vi "setSlideState.vi"(7 "Position:Top (32)":i32=32, 8 "error in (no error)":errorcluster {"code" format="Error %.0f"}, 9 "action (close)":enum16{"open", "close"}(ring)=enum."close", 10 "controlRef":refnum<vi>, 11 "paneRef":refnum<vi>) -> (0 "error out":errorcluster {"code" format="Error %.0f"}, 2 "controlRefDUP":refnum<vi>)   [LabVIEW 2017]
panel:
  out "action":enum16{"open", "close"}(ring)
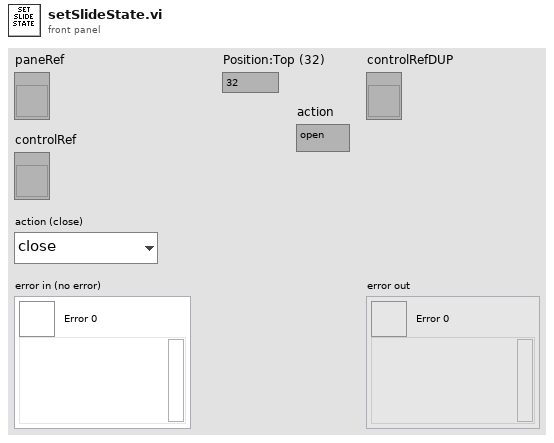
[diagram p1: front panel]
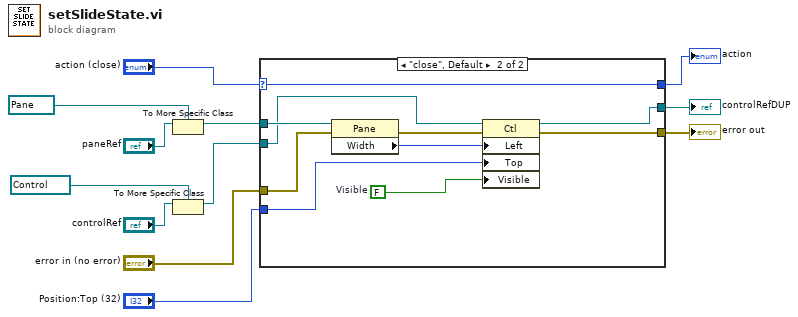
[diagram p0: block diagram]
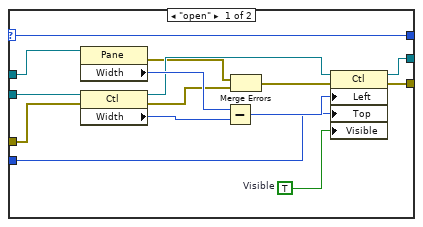
[diagram p2: hidden frame]
diagram:
  n1 = To More Specific Class(target class=refnum<vi> refnum ("paneRef 2"), reference="paneRef") -> (specific class reference=w5:refnum<vi>)  [unwired: 1 in, 1 out]
  n2 = To More Specific Class(target class=refnum<vi> refnum ("paneRef 3"), reference="controlRef") -> (specific class reference=w2:refnum<vi>)  [unwired: 1 in, 1 out]
  n3 = case shown="\"close\", Default" "action (close)" {
    selector: "action (close)" -> [w14 w29]
    tunnel: w5 -> [w27 w37]
    tunnel: w2 -> [w26 w32]
    tunnel: "error in (no error)" -> [w20 w31]
    tunnel: [w19 w35] -> w10
    tunnel: "Position:Top (32)" -> [w18 w34]
    tunnel: [w14 w29] -> w8
    tunnel: [w13 w28] -> w1
    frame "open" {
      w21 = TRUE  # Visible
      n4 = property on="Property Node" class="Pane"(reference=w27) -> (error out=w15:errorcluster, "Width"=w25:u32)  [unwired: 1 in, 1 out]
      n5 = property on="Property Node" class="Ctl"(reference=w26, error in=w20) -> (reference out=w23:refnum<vi>, error out=w16:errorcluster, "Width"=w24:u32)
      n6 = Subtract(x=w25, y=w24) -> (x-y=w22:u32)
      n7 = Merge Errors(w15, w16) -> (w17:errorcluster)
      n8 = property on="Property Node" class="Ctl"(reference=w23, error in=w17, "Left"=w22, "Top"=w18, "Visible"=w21) -> (reference out=w13:refnum<vi>, error out=w19:errorcluster)
    }
    frame "close", Default {
      w36 = FALSE  # Visible
      n9 = property on="Property Node" class="Pane"(reference=w37, error in=w31) -> (error out=w30:errorcluster, "Width"=w33:u32)  [unwired: 1 out]
      n10 = property on="Property Node" class="Ctl"(reference=w32, error in=w30, "Left"=w33, "Top"=w34, "Visible"=w36) -> (reference out=w28:refnum<vi>, error out=w35:errorcluster)
    }
  }
  "error out" <- w10
  "action" <- w8
  "controlRefDUP" <- w1
